vi "Get Method Name.vi"(11 "Message Maker in":refnum<class "Abstract Message Scripter.lvclass">) -> (2 "Method Name":string)   [LabVIEW 2020, in "Message Maker.lvlib" / "Abstract Message Scripter.lvclass"]
uses:
  Abstract Message Scripter.lvclass
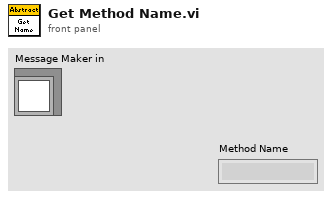
[diagram p1: front panel]
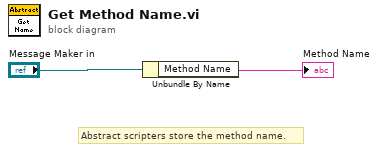
[diagram p0: block diagram]
diagram:
  # "Abstract scripters store the method name."
  n1 = Unbundle By Name("Message Maker in") -> ("Method Name"=→"Method Name":string)
